vi "POS_Back.vi"(9 "BackDistance":dbl, 11 "POS":dbl[](array[numeric])) -> (1 "Offset":dbl[](array[numeric]), 3 "POS N":dbl[](array[numeric]))   [LabVIEW 2018]
uses:
  <vilib>/Analysis/coordinate.llb/2D Cartesian Coordinate Rotation (Scalar).vi
  <vilib>/Analysis/NI_AALPro.lvlib
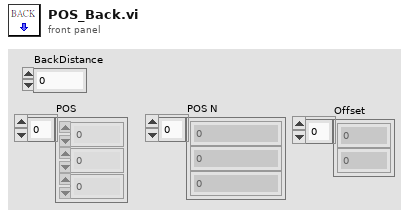
[diagram p1: front panel]
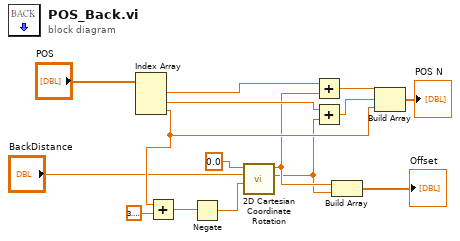
[diagram p0: block diagram]
diagram:
  n1 = Index Array(array="POS") -> (element #1=w13:dbl, element #2=w12:dbl, element #3=w8:dbl)  [unwired: 3 in]
  n2 = Add(x=w8, y=3.141592653589793) -> (x+y=w6:dbl)
  n3 = Negate(x=w6) -> (-x=w5:dbl)
  n4 = call-poly <vilib>:"2D Cartesian Coordinate Rotation.vi"("theta"=w5, "y"="BackDistance", "x"=0.0) -> ("y out"=w2:dbl, "x out"=w3:dbl)  [unwired: 6 in, 1 out]
  n5 = Add(x=w13, y=w3) -> (x+y=w10:dbl)
  n6 = Add(x=w12, y=w2) -> (x+y=w9:dbl)
  n7 = Build Array(w3, w2) -> (→"Offset":dbl[])
  n8 = Build Array(w10, w9, w8) -> (→"POS N":dbl[])
